vi "ObservadorPequeño.vi"(0 "entrada planta":dbl, 8 "salida planta":dbl, 11 "xk +1":T1=[[0.0], [0.0]]) -> (1 "Perturbacion":dbl, 2 "velocidad":dbl, 3 "xk":T1)   [LabVIEW 2018]
uses:
  <vilib>/Analysis/Matrix/Datatypes/RealMatrix.ctl
  <vilib>/Analysis/Matrix/Numeric/Conversions/Array To Matrix - RA.vi
  <vilib>/Analysis/Matrix/Numeric/Conversions/Array To Matrix - RA2.vi
  <vilib>/Analysis/Matrix/Numeric/Multiply/Multiply - RM,RM.vi
  <vilib>/Analysis/Matrix/Numeric/Add/Add - RM,RM.vi
  <vilib>/Analysis/Matrix/NI_Matrix.lvlib
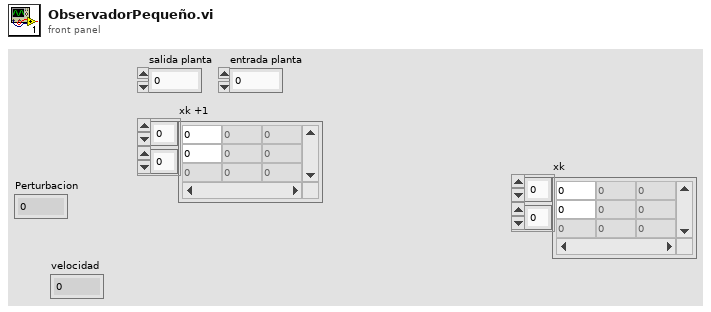
[diagram p1: front panel]
types:
  T1 = typedef "NI_Matrix.lvlib/RealMatrix.ctl" = dbl[][]
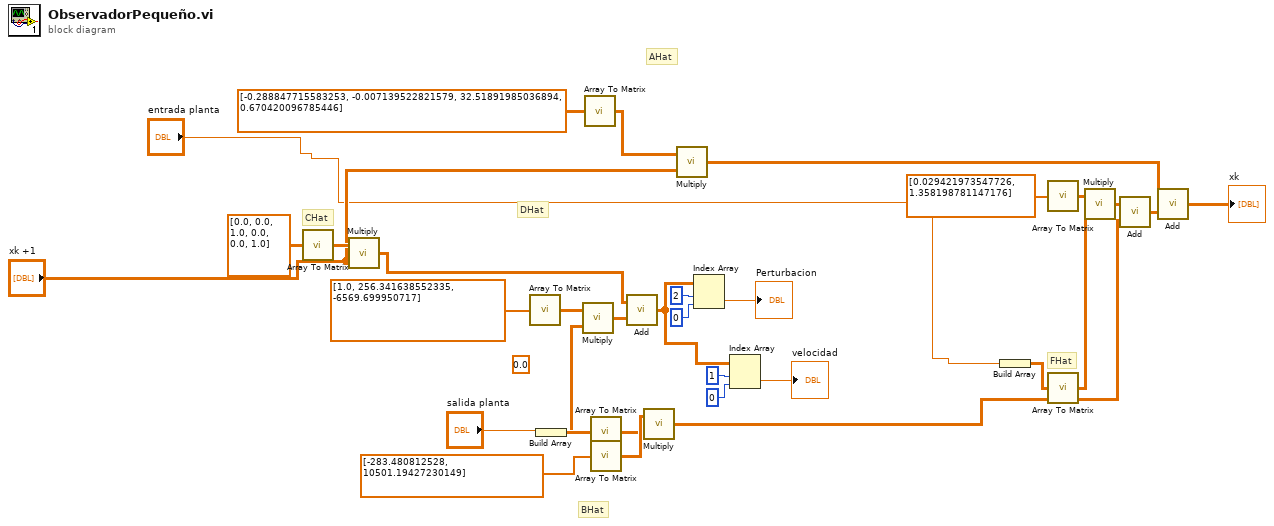
[diagram p0: block diagram]
diagram:
  (unwired) 0.0
  # "DHat"
  # "CHat"
  # "FHat"
  # "AHat"
  # "BHat"
  n1 = call-poly <vilib>:"Array To Matrix.vi"("Real 2D Array"=dbl[][] [[0.0, 0.0], [1.0, 0.0], [0.0, 1.0]]) -> ("Real Matrix"=w14:T1)
  n2 = call-poly <vilib>:"Multiply.vi"("Real Matrix B"="xk +1", "Real Matrix A"=w14) -> ("A * B"=w13:T1)
  n3 = call-poly <vilib>:"Array To Matrix.vi"("Real 1D Array"=dbl[] [1.0, 256.341638552335, -6569.699950717] ("element")) -> ("Real Matrix (Column Vector)"=w24:T1)
  n4 = Build Array("salida planta") -> (w30:T1)
  n5 = call-poly <vilib>:"Array To Matrix.vi"("Real 2D Array"=dbl[][] [[-0.288847715583253, -0.007139522821579], [32.51891985036894, 0.670420096785446]] ("element")) -> ("Real Matrix"=w23:T1)
  n6 = call-poly <vilib>:"Array To Matrix.vi"("Real 2D Array"=w30) -> ("Real Matrix"=w17:T1)
  n7 = call-poly <vilib>:"Multiply.vi"("Real Matrix B"=w17, "Real Matrix A"=w24) -> ("A * B"=w15:T1)
  n8 = call-poly <vilib>:"Array To Matrix.vi"("Real 1D Array"=dbl[] [-283.480812528, 10501.19427230149] ("element")) -> ("Real Matrix (Column Vector)"=w18:T1)
  n9 = call-poly <vilib>:"Add.vi"("Real Matrix B"=w15, "Real Matrix A"=w13) -> ("A + B"=w1:T1)
  n10 = call-poly <vilib>:"Multiply.vi"("Real Matrix B"=w17, "Real Matrix A"=w18) -> ("A * B"=w16:T1)
  n11 = call-poly <vilib>:"Multiply.vi"("Real Matrix B"="xk +1", "Real Matrix A"=w23) -> ("A * B"=w22:T1)
  n12 = Index Array(array=w1, index (row)=2, index (col)=0) -> (element=→"Perturbacion":dbl)
  n13 = Index Array(array=w1, index (row)=1, index (col)=0) -> (element=→"velocidad":dbl)
  n14 = Build Array("entrada planta") -> (w31:T1)
  n15 = call-poly <vilib>:"Array To Matrix.vi"("Real 1D Array"=dbl[] [0.029421973547726, 1.358198781147176] ("element")) -> ("Real Matrix (Column Vector)"=w21:T1)
  n16 = call-poly <vilib>:"Array To Matrix.vi"("Real 2D Array"=w31) -> ("Real Matrix"=w20:T1)
  n17 = call-poly <vilib>:"Multiply.vi"("Real Matrix B"=w20, "Real Matrix A"=w21) -> ("A * B"=w19:T1)
  n18 = call-poly <vilib>:"Add.vi"("Real Matrix B"=w16, "Real Matrix A"=w19) -> ("A + B"=w29:T1)
  n19 = call-poly <vilib>:"Add.vi"("Real Matrix B"=w29, "Real Matrix A"=w22) -> ("A + B"=→"xk":T1)
